vi "Time-calllucated_temp_graph.vi"() -> ()   [LabVIEW 2017]
uses:
  <vilib>/Utility/miscctls.llb/LVCursorListTypeDef.ctl
  <vilib>/measure/NI_MAPro.lvlib
panel:
  out "size(s) 2":i32
  out "Array 11":ext[](array[numeric])
  out "Array 8":timestamp[](array[timestamp])
  out "appended array":timestamp[][](array[timestamp])
  out "deleted portion":ext[](array[numeric])
  out "Array 10":ext[](array[numeric])
  out "Array 9":ext[][](array[numeric])
  out "Array 7":bool[](array[boolean])
  out "output cluster 3":T1(array[cluster])
  in  "Cursor List 3":T2
  out "Numeric 2":i32
  out "Array 6":timestamp[](array[timestamp])
  out "Array 5":dbl[](array[numeric])
  out "Array 4":i32[](array[numeric])
  out "Array 3":u16[](array[numeric])
  out "Array 2":u16[](array[numeric])
  out "Valley Value":dbl[](array[numeric])
  out "Valley Value index":u16[](array[numeric])
  out "Peak Value index":u16[](array[numeric])
  out "Peak Value":dbl[](array[numeric])
  out "# found 2":i32
  in  "peaks/valleys 2":u16(ring)=1 items=["Peaks", "Valleys"]
  out "x = y?":bool
  out "x+y 2":i32
  out "STOP THRESHOLD TRIGGER":i32
  out "START THRESHOLD TRIGGER":i32
  out "Array":timestamp[](array[timestamp])
  out "Numeric":i32
  out "Locations":dbl[](array[numeric]) format="%0.2f"
  out "size(s)":i32
  out "2nd Derivatives":dbl[](array[numeric]) format="%0.2f"
  out "unsigned 16bit integer":u16
  out "output cluster 2":T1(array[cluster])
  in  "Cursor List 2":T2
  out "XY Graph 3":cluster{"X":dbl, "X 2":dbl}[](graph)
  out "element":dbl
  in  "peaks/valleys":u16(ring) items=["Peaks", "Valleys"]
  in  "width":i32=3
  out "# found":i32
  in  "threshold":dbl=130.0 format="%#_13g"
  out "Y":dbl[](array[numeric]) format="%0.2f"
  out "X":dbl[](array[numeric]) format="%0.2f"
  out "time stamp":timestamp[](array[timestamp])
  out "XY Graph 2":cluster{"time stamp":timestamp, "X":dbl}[](graph)
  out "number":ext[](array[numeric])
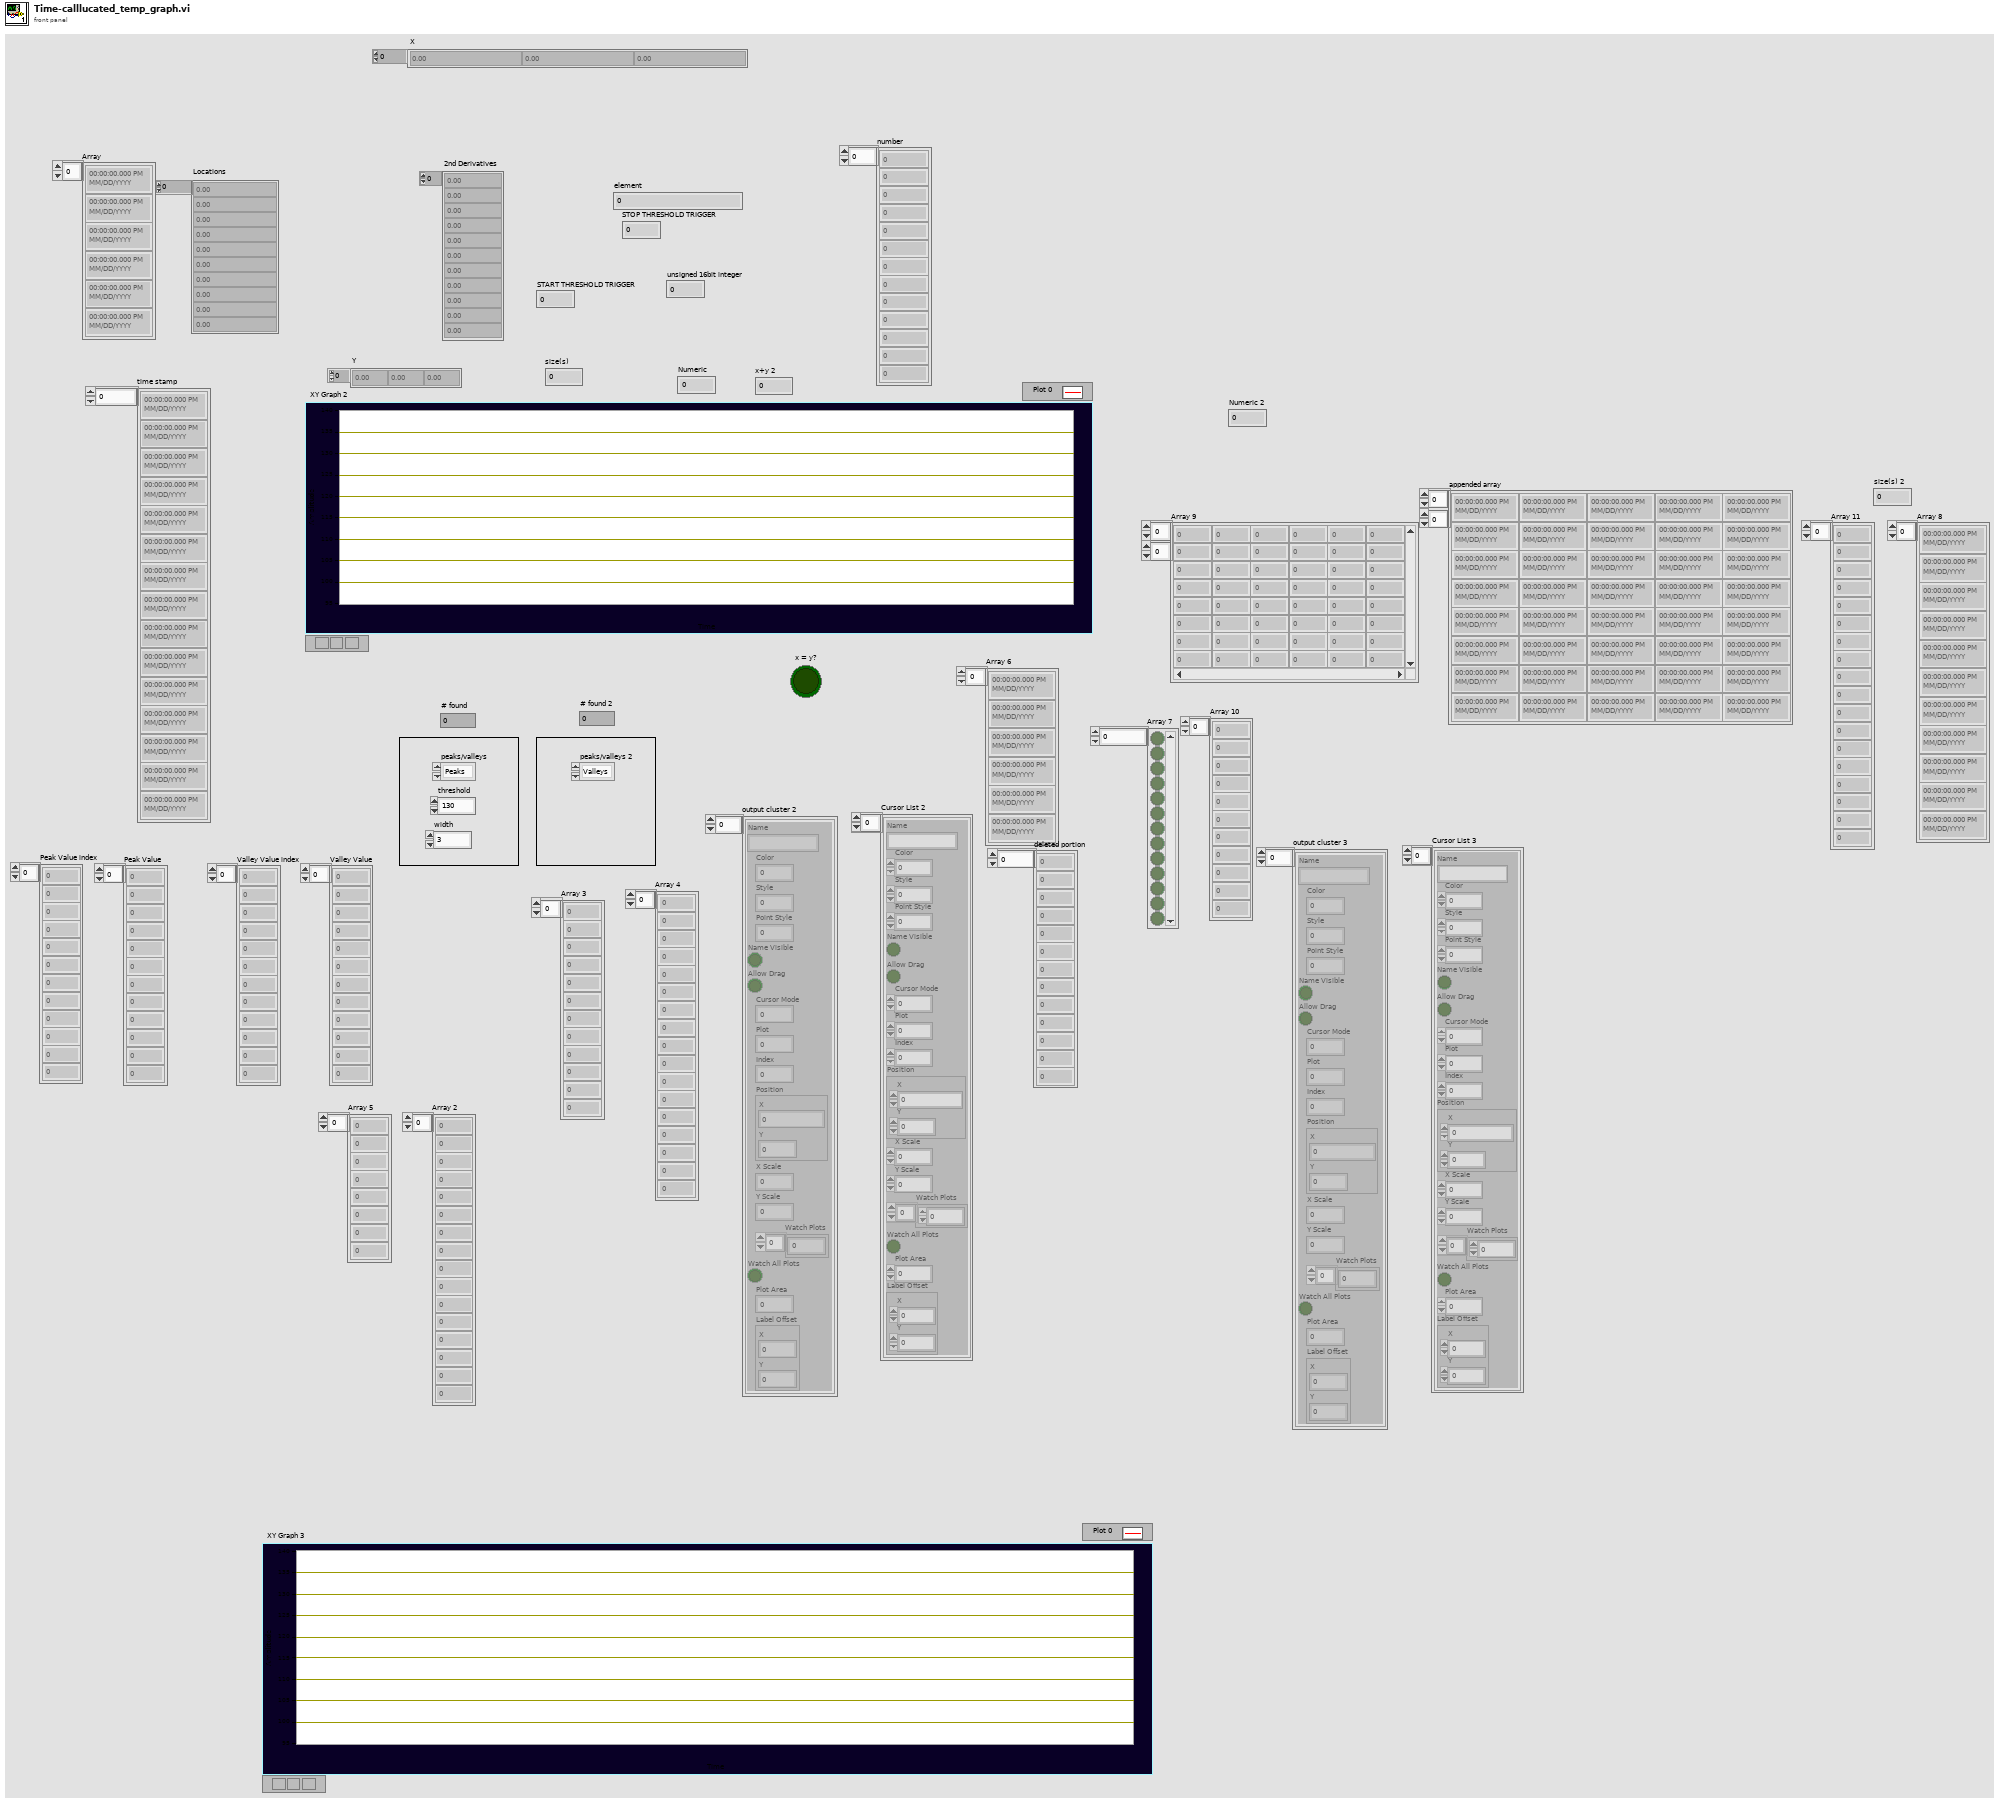
[diagram p1: front panel]
types:
  T1 = cluster{"Name":string, "Color":u32, "Style":u8, "Point Style":u8, "Name Visible":bool, "Allow Drag":bool, "Cursor Mode":u32, "Plot":i32, "Index":i32, "Position":cluster{"X":dbl, "Y":dbl}, "X Scale":u32, "Y Scale":u32, "Watch Plots":i32[], "Watch All Plots":bool, "Plot Area":i32, "Label Offset":cluster{"X":dbl, "Y":dbl}}[]
  T2 = typedef "LVCursorListTypeDef.ctl" = cluster{"Name":string, "Color":u32, "Style":u8, "Point Style":u8, "Name Visible":bool, "Allow Drag":bool, "Cursor Mode":u32, "Plot":i32, "Index":i32, "Position":cluster{"X":dbl, "Y":dbl}, "X Scale":u32, "Y Scale":u32, "Watch Plots":i32[], "Watch All Plots":bool, "Plot Area":i32, "Label Offset":cluster{"X":dbl, "Y":dbl}}[]
  T3 = typedef "LVDateTimeRec.ctl" = cluster{"fractional second":dbl, "second":i32, "minute":i32, "hour":i32, "day of month":i32, "month":i32, "year":i32, "day of week":i32, "day of year":i32, "DST":i32}
  T4 = cluster{"Name":string, "Color":u32, "Style":u8, "Point Style":u8, "Name Visible":bool, "Allow Drag":bool, "Cursor Mode":u32, "Plot":i32, "Index":i32, "Position":cluster{"X":dbl, "Y":dbl}, "X Scale":u32, "Y Scale":u32, "Watch Plots":i32[], "Watch All Plots":bool, "Plot Area":i32, "Label Offset":cluster{"X":dbl, "Y":dbl}}
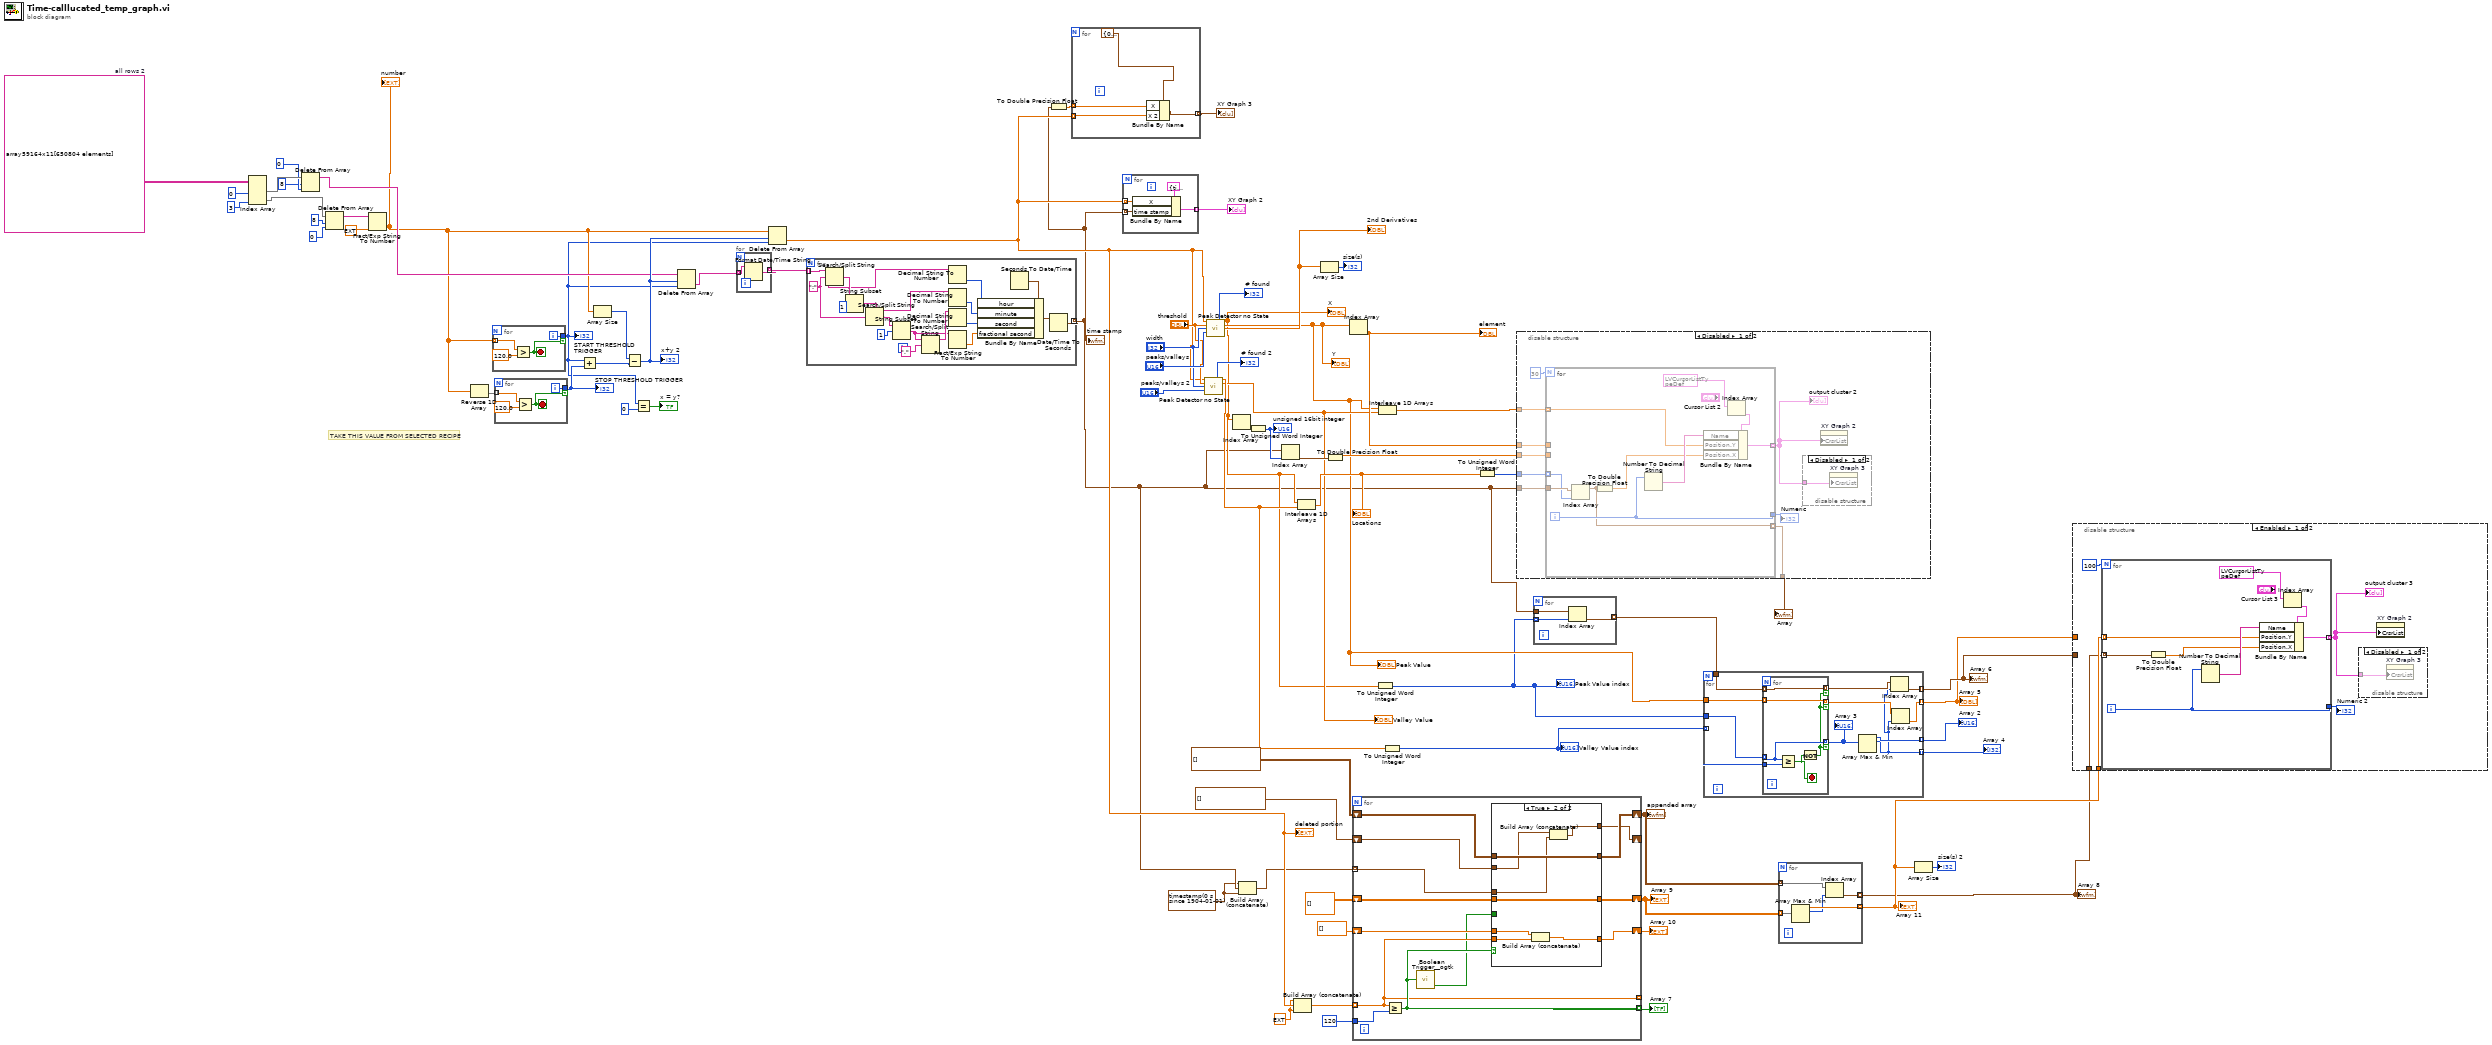
[diagram p0: block diagram]
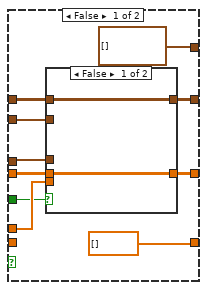
[diagram p2: hidden frame]
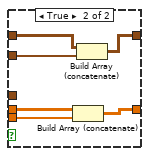
[diagram p3: hidden frame]
diagram:
  w9 = timestamp(0 s since 1904-01-01) ("time stamp")
  w11 = ext 0.0 ("String")
  w67 = string[][] array59164x11[650804 elements]  # all rows 2
  # "TAKE THIS VALUE FROM SELECTED RECIPE"
  n1 = Index Array(array=w67, index (col) #1=0 ("index (row)"), index (col) #2=3 ("disabled index (col)")) -> (element #1=w72:string[], element #2=w68:string[])  [unwired: 2 in]
  n2 = Delete From Array(array=w72, length=8 ("index (row)"), index=0 ("index (row)")) -> (array with subset deleted=w42:string[])  [unwired: 1 out]
  n3 = Delete From Array(array=w68, length=8 ("index (row)"), index=0 ("index (row)")) -> (array with subset deleted=w49:string[])  [unwired: 1 out]
  n4 = Fract/Exp String To Number(string=w49, default (0 dbl)=ext 0.0 ("String")) -> (number=w40:ext[])  [unwired: 2 in, 1 out]
  "number" <- w40
  n5 = Reverse 1D Array(array=w40) -> (reversed array=w48:ext[])
  n6 = for {
    tunnel: w40 -> [w75] mode=indexing
    tunnel: [w74] -> w39 if=w73
    i -> [w74]
    stop <- w73 stop-if-true
    n7 = Greater?(x=w75, y=120.0) -> (0:w73:bool)
  }
  "START THRESHOLD TRIGGER" <- w39
  n8 = for {
    tunnel: w48 -> [w79] mode=indexing
    tunnel: [w78] -> w47 if=w77
    i -> [w78]
    stop <- w77 stop-if-true
    n9 = Greater?(x=w79, y=120.0) -> (0:w77:bool)
  }
  "STOP THRESHOLD TRIGGER" <- w47
  n10 = Add(x=w39, y=w47) -> (x+y=w45:i32)
  n11 = Array Size(array=w40) -> (size(s)=w46:i32)
  n12 = Subtract(x=w46, y=w45) -> (x-y=w44:i32)
  "x+y 2" <- w44
  n13 = Equal?(x=w39, y=0) -> (x = y?=→"x = y?":bool)
  n14 = Delete From Array(array=w42, length=w44, index=w39) -> (deleted portion=w43:string[])  [unwired: 1 out]
  n15 = for {
    tunnel: w43 -> [w82] mode=indexing
    tunnel: [w81] -> w63 mode=indexing
    n16 = Format Date/Time String(time format string (%c)=w82) -> (date/time string=w81:string)  [unwired: 2 in]
  }
  n17 = Delete From Array(array=w40, length=w44, index=w39) -> (deleted portion=w13:ext[])  [unwired: 1 out]
  "deleted portion" <- w13
  n18 = for {
    tunnel: w63 -> [w91] mode=indexing
    tunnel: [w99] -> w10 mode=indexing
    w98 = ":" ("format string")
    n19 = Search/Split String(string=w91, search string/char (-)=w98) -> (substring before match=w87:string, match + rest of string=w96:string)  [unwired: 1 in, 1 out]
    n20 = String Subset(string=w96, offset (0)=1) -> (substring=w95:string)  [unwired: 1 in]
    n21 = Search/Split String(string=w95, search string/char (-)=w98) -> (substring before match=w86:string, match + rest of string=w93:string)  [unwired: 1 in, 1 out]
    n22 = String Subset(string=w93, offset (0)=1) -> (substring=w85:string)  [unwired: 1 in]
    n23 = Search/Split String(string=w85, search string/char (-)="." ("format string")) -> (substring before match=w90:string)  [unwired: 1 in, 2 out]
    n24 = Decimal String To Number(string=w87) -> (number=w88:i32)  [unwired: 2 in, 1 out]
    n25 = Decimal String To Number(string=w86) -> (number=w89:i32)  [unwired: 2 in, 1 out]
    n26 = Decimal String To Number(string=w90) -> (number=w83:i32)  [unwired: 2 in, 1 out]
    n27 = Fract/Exp String To Number(string=w85) -> (number=w84:dbl)  [unwired: 3 in, 1 out]
    n28 = Seconds To Date/Time() -> (date time rec=w100:T3)  [unwired: 2 in]
    n29 = Bundle By Name(cluster=w100, "hour"=w88, "minute"=w89, "second"=w83, "fractional second"=w84) -> (w101:T3)
    n30 = Date/Time To Seconds(2:w101) -> (0:w99:timestamp)  [unwired: 1 in]
  }
  "time stamp" <- w10
  n31 = To Double Precision Float(number=w10) -> (double precision float=w57:dbl[])
  n32 = for {
    tunnel: w57 -> [w103] mode=indexing
    tunnel: [w105] -> w56 mode=indexing
    tunnel: w13 -> [w104] mode=indexing
    n33 = Bundle By Name(cluster=cluster{"X":dbl, "X 2":dbl} {"X"=0.0, "X 2"=0.0}, "X"=w103, "X 2"=w104) -> (w105:cluster{"X":dbl, "X 2":dbl})
  }
  "XY Graph 3" <- w56
  n34 = for {
    tunnel: w13 -> [w106] mode=indexing
    tunnel: [w109] -> w59 mode=indexing
    tunnel: w10 -> [w107] mode=indexing
    n35 = Bundle By Name(cluster=cluster{"time stamp":timestamp, "X":dbl} {"time stamp"=timestamp(0 s since 1904-01-01), "X"=0.0}, "X"=w106, "time stamp"=w107) -> (w109:cluster{"time stamp":timestamp, "X":dbl})
  }
  "XY Graph 2" <- w59
  n36 = call <vilib>:"Peak Detector no State.vi"("X"=w13, "threshold"="threshold", "width"="width", "peaks/valleys"="peaks/valleys 2") -> ("# found"=→"# found 2":i32, "Locations"=w29:dbl[], "Amplitudes"=w28:dbl[])  [unwired: 4 in, 5 out]
  "Valley Value" <- w28
  n37 = call <vilib>:"Peak Detector no State.vi"("X"=w13, "threshold"="threshold", "width"="width", "peaks/valleys"="peaks/valleys") -> ("# found"=→"# found":i32, "Locations"=w19:dbl[], "Amplitudes"=w24:dbl[], "2nd Derivatives"=w52:dbl[])  [unwired: 4 in, 4 out]
  "X" <- w19
  "Y" <- w24
  "2nd Derivatives" <- w52
  "Peak Value" <- w24
  n38 = Index Array(array=w19) -> (element=w55:dbl)  [unwired: 1 in]
  n39 = Build Array (concatenate)(w9, w10, w9) -> (w6:timestamp[])
  n40 = To Unsigned Word Integer(number=w55) -> (unsigned 16bit integer=w54:u16)
  "unsigned 16bit integer" <- w54
  n41 = Index Array(array=w10, index=w54) -> (element=w58:timestamp)
  n42 = Build Array (concatenate)(w11, w13, w11) -> (w12:ext[])
  n43 = Interleave 1D Arrays(w19, w29) -> (w32:dbl[])
  "Locations" <- w32
  n44 = Array Size(array=w52) -> (size(s)=→"size(s)":i32)
  n45 = To Double Precision Float(number=w58) -> (double precision float=w41:dbl)
  n46 = Index Array(array=w24) -> (element=w53:dbl)  [unwired: 1 in]
  "element" <- w53
  n47 = for {
    tunnel: w12 -> [w120] mode=indexing
    tunnel: [w121] -> w17 mode=indexing
    tunnel: 120 -> [w122]
    tunnel: [w120] -> _ mode=indexing
    shift-right: [w119] -> w14
    shift-left: ext[] [] -> [w118]
    shift-right: [w116] -> w5
    shift-left: ext[][] [] -> [w117]
    tunnel: w6 -> [w114] mode=indexing
    shift-right: [w113] -> w4
    shift-left: timestamp[][] [] ("appended array") -> [w112]
    shift-right: [w110] -> _
    shift-left: timestamp[] [] ("appended array") -> [w111]
    n48 = Greater Or Equal?(x=w120, y=w122) -> (x >= y?=w121:bool)
    n49 = call <userlib>:"Boolean Trigger__ogtk.vi"("Boolean Input"=w121) -> ("Falling Edge"=w115:bool)  [unwired: 1 in, 1 out]
    n50 = case shown="True" w121 {
      tunnel: w120 -> [_ w148]
      tunnel: [ext[] [] w147] -> w119
      tunnel: w118 -> [w129 w145]
      tunnel: w117 -> [w130 w146]
      tunnel: [w131 w146] -> w116
      tunnel: w115 -> [w128 _]
      tunnel: w114 -> [w127 w141]
      tunnel: [w126 w144] -> w113
      tunnel: w112 -> [w125 w144]
      tunnel: w111 -> [w124 w142]
      tunnel: [timestamp[] [] ("appended array") w143] -> w110
      frame False {
        n51 = case shown="False" w128 {
          tunnel: [w134 w140] -> w131
          tunnel: w130 -> [w134 w139]
          tunnel: w129 -> [_ w138]
          tunnel: w127 -> [_ _]
          tunnel: [w133 w137] -> w126
          tunnel: w125 -> [w133 w136]
          tunnel: w124 -> [_ w135]
          frame False {
          }
          frame True {
            n52 = Build Array (concatenate)(w139, w138) -> (w140:ext[][])
            n53 = Build Array (concatenate)(w136, w135) -> (w137:timestamp[][])
          }
        }
      }
      frame True {
        n54 = Build Array (concatenate)(w145, w148) -> (w147:ext[])
        n55 = Build Array (concatenate)(w142, w141) -> (w143:timestamp[])
      }
    }
  }
  "Array 7" <- w17
  "Array 9" <- w5
  "Array 10" <- w14
  "appended array" <- w4
  n56 = To Unsigned Word Integer(number=w19) -> (unsigned 16bit integer=w21:u16[])
  "Peak Value index" <- w21
  n57 = Interleave 1D Arrays(w24, w28) -> (w31:dbl[])
  n58 = To Unsigned Word Integer(number=w29) -> (unsigned 16bit integer=w27:u16[])
  "Valley Value index" <- w27
  n59 = To Unsigned Word Integer(number=w32) -> (unsigned 16bit integer=w30:u16[])
  n60 = disable-structure shown="Disabled" {
    disable-tunnel: w41 -> [w157 _]
    disable-tunnel: w53 -> [w156 _]
    disable-tunnel: w31 -> [w150 _]
    disable-tunnel: w10 -> [w155 _]
    disable-tunnel: w30 -> [w149 _]
    disable-tunnel: [w153 _] -> w50
    frame Disabled {
      n61 = for {
        N: 30 -> [_]
        tunnel: [w167] -> w151 mode=indexing
        tunnel: w157 -> [_]
        tunnel: w156 -> [_]
        tunnel: w150 -> [w165] mode=indexing
        tunnel: w155 -> [w163]
        tunnel: w149 -> [w162] mode=indexing
        tunnel: [w161] -> w154
        tunnel: [w160] -> w153 mode=indexing
        i -> [w161]
        n62 = Index Array(array=w163, index=w162) -> (element=w160:timestamp)
        n63 = To Double Precision Float(number=w160) -> (double precision float=w164:dbl)
        n64 = Number To Decimal String(number=w161) -> (decimal integer string=w166:string)  [unwired: 1 in]
        n65 = Index Array(array=T2 [{"Name"="0", "Color"=0, "Style"=0, "Point Style"=13, "Name Visible"=FALSE, "Allow Drag"=FALSE, "Cursor Mode"=0, "Plot"=0, "Index"=0, "Position"={"X"=3725289003.72, "Y"=121.765}, "X Scale"=0, "Y Scale"=0, "Watch Plots"=[], "Watch All Plots"=FALSE, "Plot Area"=0, "Label Offset"={"X"=0.0, "Y"=0.0}}, {"Name"="1", "Color"=0, "Style"=0, "Point Style"=0, "Name Visible"=FALSE, "Allow Drag"=FALSE, "Cursor Mode"=0, "Plot"=0, "Index"=0, "Position"={"X"=3725289003.725, "Y"=125.02090909090909}, "X Scale"=0, "Y Scale"=0, "Watch Plots"=[], "Watch All Plots"=FALSE, "Plot Area"=0, "Label Offset"={"X"=0.0, "Y"=0.0}}, {"Name"="2", "Color"=0, "Style"=0, "Point Style"=0, "Name Visible"=FALSE, "Allow Drag"=FALSE, "Cursor Mode"=0, "Plot"=0, "Index"=0, "Position"={"X"=3725289003.728, "Y"=128.01}, "X Scale"=0, "Y Scale"=0, "Watch Plots"=[], "Watch All Plots"=FALSE, "Plot Area"=0, "Label Offset"={"X"=0.0, "Y"=0.0}}, {"Name"="3", "Color"=0, "Style"=0, "Point Style"=0, "Name Visible"=FALSE, "Allow Drag"=FALSE, "Cursor Mode"=0, "Plot"=0, "Index"=0, "Position"={"X"=3725289003.73, "Y"=123.4901219512195}, "X Scale"=0, "Y Scale"=0, "Watch Plots"=[], "Watch All Plots"=FALSE, "Plot Area"=0, "Label Offset"={"X"=0.0, "Y"=0.0}}, {"Name"="4", "Color"=0, "Style"=0, "Point Style"=0, "Name Visible"=FALSE, "Allow Drag"=FALSE, "Cursor Mode"=0, "Plot"=0, "Index"=0, "Position"={"X"=3725289003.732, "Y"=120.435}, "X Scale"=0, "Y Scale"=0, "Watch Plots"=[], "Watch All Plots"=FALSE, "Plot Area"=0, "Label Offset"={"X"=0.0, "Y"=0.0}}, {"Name"="5", "Color"=0, "Style"=0, "Point Style"=0, "Name Visible"=FALSE, "Allow Drag"=FALSE, "Cursor Mode"=0, "Plot"=0, "Index"=0, "Position"={"X"=3725289003.752, "Y"=121.25480392156864}, "X Scale"=0, "Y Scale"=0, "Watch Plots"=[], "Watch All Plots"=FALSE, "Plot Area"=0, "Label Offset"={"X"=0.0, "Y"=0.0}}, {"Name"="6", "Color"=0, "Style"=0, "Point Style"=0, "Name Visible"=FALSE, "Allow Drag"=FALSE, "Cursor Mode"=0, "Plot"=0, "Index"=0, "Position"={"X"=3725289003.756, "Y"=123.92999999999999}, "X Scale"=0, "Y Scale"=0, "Watch Plots"=[], "Watch All Plots"=FALSE, "Plot Area"=0, "Label Offset"={"X"=0.0, "Y"=0.0}}, {"Name"="7", "Color"=0, "Style"=0, "Point Style"=0, "Name Visible"=FALSE, "Allow Drag"=FALSE, "Cursor Mode"=0, "Plot"=0, "Index"=0, "Position"={"X"=3725289003.762, "Y"=127.01970588235294}, "X Scale"=0, "Y Scale"=0, "Watch Plots"=[], "Watch All Plots"=FALSE, "Plot Area"=0, "Label Offset"={"X"=0.0, "Y"=0.0}}, {"Name"="8", "Color"=0, "Style"=0, "Point Style"=0, "Name Visible"=FALSE, "Allow Drag"=FALSE, "Cursor Mode"=0, "Plot"=0, "Index"=0, "Position"={"X"=3725289003.765, "Y"=131.29425531914893}, "X Scale"=0, "Y Scale"=0, "Watch Plots"=[], "Watch All Plots"=FALSE, "Plot Area"=0, "Label Offset"={"X"=0.0, "Y"=0.0}}, {"Name"="9", "Color"=0, "Style"=0, "Point Style"=0, "Name Visible"=FALSE, "Allow Drag"=FALSE, "Cursor Mode"=0, "Plot"=0, "Index"=0, "Position"={"X"=3725289003.767, "Y"=128.4116891891892}, "X Scale"=0, "Y Scale"=0, "Watch Plots"=[], "Watch All Plots"=FALSE, "Plot Area"=0, "Label Offset"={"X"=0.0, "Y"=0.0}}, {"Name"="10", "Color"=0, "Style"=0, "Point Style"=0, "Name Visible"=FALSE, "Allow Drag"=FALSE, "Cursor Mode"=0, "Plot"=0, "Index"=0, "Position"={"X"=3725289003.768, "Y"=122.84}, "X Scale"=0, "Y Scale"=0, "Watch Plots"=[], "Watch All Plots"=FALSE, "Plot Area"=0, "Label Offset"={"X"=0.0, "Y"=0.0}}, {"Name"="11", "Color"=0, "Style"=0, "Point Style"=0, "Name Visible"=FALSE, "Allow Drag"=FALSE, "Cursor Mode"=0, "Plot"=0, "Index"=0, "Position"={"X"=3725289003.794, "Y"=121.99}, "X Scale"=0, "Y Scale"=0, "Watch Plots"=[], "Watch All Plots"=FALSE, "Plot Area"=0, "Label Offset"={"X"=0.0, "Y"=0.0}}, {"Name"="12", "Color"=0, "Style"=0, "Point Style"=0, "Name Visible"=FALSE, "Allow Drag"=FALSE, "Cursor Mode"=0, "Plot"=0, "Index"=0, "Position"={"X"=3725289003.803, "Y"=128.6199504950495}, "X Scale"=0, "Y Scale"=0, "Watch Plots"=[], "Watch All Plots"=FALSE, "Plot Area"=0, "Label Offset"={"X"=0.0, "Y"=0.0}}, {"Name"="13", "Color"=0, "Style"=0, "Point Style"=0, "Name Visible"=FALSE, "Allow Drag"=FALSE, "Cursor Mode"=0, "Plot"=0, "Index"=0, "Position"={"X"=3725289003.806, "Y"=132.86499999999998}, "X Scale"=0, "Y Scale"=0, "Watch Plots"=[], "Watch All Plots"=FALSE, "Plot Area"=0, "Label Offset"={"X"=0.0, "Y"=0.0}}, {"Name"="14", "Color"=0, "Style"=0, "Point Style"=0, "Name Visible"=FALSE, "Allow Drag"=FALSE, "Cursor Mode"=0, "Plot"=0, "Index"=0, "Position"={"X"=3725289003.808, "Y"=128.93437743190663}, "X Scale"=0, "Y Scale"=0, "Watch Plots"=[], "Watch All Plots"=FALSE, "Plot Area"=0, "Label Offset"={"X"=0.0, "Y"=0.0}}, {"Name"="15", "Color"=0, "Style"=0, "Point Style"=0, "Name Visible"=FALSE, "Allow Drag"=FALSE, "Cursor Mode"=0, "Plot"=0, "Index"=0, "Position"={"X"=3725289003.83, "Y"=121.8}, "X Scale"=0, "Y Scale"=0, "Watch Plots"=[], "Watch All Plots"=FALSE, "Plot Area"=0, "Label Offset"={"X"=0.0, "Y"=0.0}}, {"Name"="16", "Color"=0, "Style"=0, "Point Style"=0, "Name Visible"=FALSE, "Allow Drag"=FALSE, "Cursor Mode"=0, "Plot"=0, "Index"=0, "Position"={"X"=3725289003.84, "Y"=128.54500000000002}, "X Scale"=0, "Y Scale"=0, "Watch Plots"=[], "Watch All Plots"=FALSE, "Plot Area"=0, "Label Offset"={"X"=0.0, "Y"=0.0}}, {"Name"="17", "Color"=0, "Style"=0, "Point Style"=0, "Name Visible"=FALSE, "Allow Drag"=FALSE, "Cursor Mode"=0, "Plot"=0, "Index"=0, "Position"={"X"=3725289003.842, "Y"=129.14884615384614}, "X Scale"=0, "Y Scale"=0, "Watch Plots"=[], "Watch All Plots"=FALSE, "Plot Area"=0, "Label Offset"={"X"=0.0, "Y"=0.0}}, {"Name"="18", "Color"=0, "Style"=0, "Point Style"=0, "Name Visible"=FALSE, "Allow Drag"=FALSE, "Cursor Mode"=0, "Plot"=0, "Index"=0, "Position"={"X"=3725289003.845, "Y"=133.010296912114}, "X Scale"=0, "Y Scale"=0, "Watch Plots"=[], "Watch All Plots"=FALSE, "Plot Area"=0, "Label Offset"={"X"=0.0, "Y"=0.0}}, {"Name"="19", "Color"=0, "Style"=0, "Point Style"=0, "Name Visible"=FALSE, "Allow Drag"=FALSE, "Cursor Mode"=0, "Plot"=0, "Index"=0, "Position"={"X"=3725289003.847, "Y"=128.22329145728645}, "X Scale"=0, "Y Scale"=0, "Watch Plots"=[], "Watch All Plots"=FALSE, "Plot Area"=0, "Label Offset"={"X"=0.0, "Y"=0.0}}] ("Cursor List")) -> (element=w168:T4)  [unwired: 1 in]
        n66 = Bundle By Name(cluster=w168, "Name"=w166, "Position.Y"=w165, "Position.X"=w164) -> (w167:T4)
      }
      "output cluster 2" <- w151
      "Numeric" <- w154
      n67 = disable-structure shown="Disabled" {
        disable-tunnel: w151 -> [w158 _]
        frame Disabled {
          n68 = property on="XY Graph 3" class="XYGraph (strict)"("CrsrList"=w158) -> ()  [unwired: 2 in, 2 out]
        }
        frame Enabled {
        }
      }
      n69 = property on="XY Graph 2" class="XYGraph (strict)"("CrsrList"=w151) -> ()  [unwired: 2 in, 2 out]
    }
    frame Enabled {
    }
  }
  "Array" <- w50
  n70 = for {
    tunnel: w10 -> [w171]
    tunnel: w21 -> [w170] mode=indexing
    tunnel: [w169] -> w20 mode=indexing
    n71 = Index Array(array=w171, index=w170) -> (element=w169:timestamp)
  }
  n72 = for {
    tunnel: w27 -> [w181] mode=indexing
    tunnel: w21 -> [w182]
    tunnel: [w179] -> w26 mode=indexing
    tunnel: [w173] -> w25 mode=indexing
    tunnel: w24 -> [w178]
    tunnel: [w176] -> w22 mode=indexing
    tunnel: w20 -> [w175]
    tunnel: [w172] -> w23 mode=indexing
    n73 = for {
      tunnel: w181 -> [w188]
      tunnel: w182 -> [w187] mode=indexing
      tunnel: [w187] -> w180 mode=indexing if=w183
      tunnel: [w185] -> w177 mode=indexing if=w183
      tunnel: w178 -> [w185] mode=indexing
      tunnel: w175 -> [w184] mode=indexing
      tunnel: [w184] -> w174 mode=indexing if=w183
      stop <- w186 stop-if-true
      n74 = Greater Or Equal?(x=w187, y=w188) -> (x >= y?=w186:bool)
      n75 = Not(x=w186) -> (.not. x?=w183:bool)
    }
    "Array 3" <- w180
    n76 = Array Max & Min(array=w180) -> (max value=w179:u16, max index (indices)=w173:i32)  [unwired: 2 out]
    n77 = Index Array(array=w174, index=w173) -> (element=w172:timestamp)
    n78 = Index Array(array=w177, index=w173) -> (element=w176:dbl)
  }
  "Array 2" <- w26
  "Array 4" <- w25
  "Array 5" <- w22
  "Array 6" <- w23
  n79 = for {
    tunnel: w5 -> [w193] mode=indexing
    tunnel: w4 -> [w191] mode=indexing
    tunnel: [w192] -> w2 mode=indexing
    tunnel: [w189] -> w1 mode=indexing
    n80 = Array Max & Min(array=w193) -> (max value=w192:ext, max index (indices)=w190:i32)  [unwired: 2 out]
    n81 = Index Array(array=w191, index=w190) -> (element=w189:timestamp)
  }
  "Array 8" <- w1
  "Array 11" <- w2
  n82 = Array Size(array=w2) -> (size(s)=→"size(s) 2":i32)
  n83 = disable-structure shown="Enabled" {
    disable-tunnel: w23 -> [_ _]
    disable-tunnel: w22 -> [_ _]
    disable-tunnel: w2 -> [w195 _]
    disable-tunnel: w1 -> [w194 _]
    frame Enabled {
      n84 = for {
        N: 100 -> [_]
        tunnel: [w206] -> w196 mode=indexing
        tunnel: [w203] -> w198
        tunnel: w194 -> [w201] mode=indexing
        tunnel: w195 -> [w200] mode=indexing
        i -> [w203]
        n85 = To Double Precision Float(number=w201) -> (double precision float=w204:dbl)
        n86 = Number To Decimal String(number=w203) -> (decimal integer string=w205:string)  [unwired: 1 in]
        n87 = Index Array(array=T2 [{"Name"="0", "Color"=0, "Style"=0, "Point Style"=13, "Name Visible"=FALSE, "Allow Drag"=FALSE, "Cursor Mode"=0, "Plot"=0, "Index"=0, "Position"={"X"=3725289003.72, "Y"=121.765}, "X Scale"=0, "Y Scale"=0, "Watch Plots"=[], "Watch All Plots"=FALSE, "Plot Area"=0, "Label Offset"={"X"=0.0, "Y"=0.0}}, {"Name"="1", "Color"=0, "Style"=0, "Point Style"=0, "Name Visible"=FALSE, "Allow Drag"=FALSE, "Cursor Mode"=0, "Plot"=0, "Index"=0, "Position"={"X"=3725289003.725, "Y"=125.02090909090909}, "X Scale"=0, "Y Scale"=0, "Watch Plots"=[], "Watch All Plots"=FALSE, "Plot Area"=0, "Label Offset"={"X"=0.0, "Y"=0.0}}, {"Name"="2", "Color"=0, "Style"=0, "Point Style"=0, "Name Visible"=FALSE, "Allow Drag"=FALSE, "Cursor Mode"=0, "Plot"=0, "Index"=0, "Position"={"X"=3725289003.728, "Y"=128.01}, "X Scale"=0, "Y Scale"=0, "Watch Plots"=[], "Watch All Plots"=FALSE, "Plot Area"=0, "Label Offset"={"X"=0.0, "Y"=0.0}}, {"Name"="3", "Color"=0, "Style"=0, "Point Style"=0, "Name Visible"=FALSE, "Allow Drag"=FALSE, "Cursor Mode"=0, "Plot"=0, "Index"=0, "Position"={"X"=3725289003.73, "Y"=123.4901219512195}, "X Scale"=0, "Y Scale"=0, "Watch Plots"=[], "Watch All Plots"=FALSE, "Plot Area"=0, "Label Offset"={"X"=0.0, "Y"=0.0}}, {"Name"="4", "Color"=0, "Style"=0, "Point Style"=0, "Name Visible"=FALSE, "Allow Drag"=FALSE, "Cursor Mode"=0, "Plot"=0, "Index"=0, "Position"={"X"=3725289003.732, "Y"=120.435}, "X Scale"=0, "Y Scale"=0, "Watch Plots"=[], "Watch All Plots"=FALSE, "Plot Area"=0, "Label Offset"={"X"=0.0, "Y"=0.0}}, {"Name"="5", "Color"=0, "Style"=0, "Point Style"=0, "Name Visible"=FALSE, "Allow Drag"=FALSE, "Cursor Mode"=0, "Plot"=0, "Index"=0, "Position"={"X"=3725289003.752, "Y"=121.25480392156864}, "X Scale"=0, "Y Scale"=0, "Watch Plots"=[], "Watch All Plots"=FALSE, "Plot Area"=0, "Label Offset"={"X"=0.0, "Y"=0.0}}, {"Name"="6", "Color"=0, "Style"=0, "Point Style"=0, "Name Visible"=FALSE, "Allow Drag"=FALSE, "Cursor Mode"=0, "Plot"=0, "Index"=0, "Position"={"X"=3725289003.756, "Y"=123.92999999999999}, "X Scale"=0, "Y Scale"=0, "Watch Plots"=[], "Watch All Plots"=FALSE, "Plot Area"=0, "Label Offset"={"X"=0.0, "Y"=0.0}}, {"Name"="7", "Color"=0, "Style"=0, "Point Style"=0, "Name Visible"=FALSE, "Allow Drag"=FALSE, "Cursor Mode"=0, "Plot"=0, "Index"=0, "Position"={"X"=3725289003.762, "Y"=127.01970588235294}, "X Scale"=0, "Y Scale"=0, "Watch Plots"=[], "Watch All Plots"=FALSE, "Plot Area"=0, "Label Offset"={"X"=0.0, "Y"=0.0}}, {"Name"="8", "Color"=0, "Style"=0, "Point Style"=0, "Name Visible"=FALSE, "Allow Drag"=FALSE, "Cursor Mode"=0, "Plot"=0, "Index"=0, "Position"={"X"=3725289003.765, "Y"=131.29425531914893}, "X Scale"=0, "Y Scale"=0, "Watch Plots"=[], "Watch All Plots"=FALSE, "Plot Area"=0, "Label Offset"={"X"=0.0, "Y"=0.0}}, {"Name"="9", "Color"=0, "Style"=0, "Point Style"=0, "Name Visible"=FALSE, "Allow Drag"=FALSE, "Cursor Mode"=0, "Plot"=0, "Index"=0, "Position"={"X"=3725289003.767, "Y"=128.4116891891892}, "X Scale"=0, "Y Scale"=0, "Watch Plots"=[], "Watch All Plots"=FALSE, "Plot Area"=0, "Label Offset"={"X"=0.0, "Y"=0.0}}, {"Name"="10", "Color"=0, "Style"=0, "Point Style"=0, "Name Visible"=FALSE, "Allow Drag"=FALSE, "Cursor Mode"=0, "Plot"=0, "Index"=0, "Position"={"X"=3725289003.768, "Y"=122.84}, "X Scale"=0, "Y Scale"=0, "Watch Plots"=[], "Watch All Plots"=FALSE, "Plot Area"=0, "Label Offset"={"X"=0.0, "Y"=0.0}}, {"Name"="11", "Color"=0, "Style"=0, "Point Style"=0, "Name Visible"=FALSE, "Allow Drag"=FALSE, "Cursor Mode"=0, "Plot"=0, "Index"=0, "Position"={"X"=3725289003.794, "Y"=121.99}, "X Scale"=0, "Y Scale"=0, "Watch Plots"=[], "Watch All Plots"=FALSE, "Plot Area"=0, "Label Offset"={"X"=0.0, "Y"=0.0}}, {"Name"="12", "Color"=0, "Style"=0, "Point Style"=0, "Name Visible"=FALSE, "Allow Drag"=FALSE, "Cursor Mode"=0, "Plot"=0, "Index"=0, "Position"={"X"=3725289003.803, "Y"=128.6199504950495}, "X Scale"=0, "Y Scale"=0, "Watch Plots"=[], "Watch All Plots"=FALSE, "Plot Area"=0, "Label Offset"={"X"=0.0, "Y"=0.0}}, {"Name"="13", "Color"=0, "Style"=0, "Point Style"=0, "Name Visible"=FALSE, "Allow Drag"=FALSE, "Cursor Mode"=0, "Plot"=0, "Index"=0, "Position"={"X"=3725289003.806, "Y"=132.86499999999998}, "X Scale"=0, "Y Scale"=0, "Watch Plots"=[], "Watch All Plots"=FALSE, "Plot Area"=0, "Label Offset"={"X"=0.0, "Y"=0.0}}, {"Name"="14", "Color"=0, "Style"=0, "Point Style"=0, "Name Visible"=FALSE, "Allow Drag"=FALSE, "Cursor Mode"=0, "Plot"=0, "Index"=0, "Position"={"X"=3725289003.808, "Y"=128.93437743190663}, "X Scale"=0, "Y Scale"=0, "Watch Plots"=[], "Watch All Plots"=FALSE, "Plot Area"=0, "Label Offset"={"X"=0.0, "Y"=0.0}}, {"Name"="15", "Color"=0, "Style"=0, "Point Style"=0, "Name Visible"=FALSE, "Allow Drag"=FALSE, "Cursor Mode"=0, "Plot"=0, "Index"=0, "Position"={"X"=3725289003.83, "Y"=121.8}, "X Scale"=0, "Y Scale"=0, "Watch Plots"=[], "Watch All Plots"=FALSE, "Plot Area"=0, "Label Offset"={"X"=0.0, "Y"=0.0}}, {"Name"="16", "Color"=0, "Style"=0, "Point Style"=0, "Name Visible"=FALSE, "Allow Drag"=FALSE, "Cursor Mode"=0, "Plot"=0, "Index"=0, "Position"={"X"=3725289003.84, "Y"=128.54500000000002}, "X Scale"=0, "Y Scale"=0, "Watch Plots"=[], "Watch All Plots"=FALSE, "Plot Area"=0, "Label Offset"={"X"=0.0, "Y"=0.0}}, {"Name"="17", "Color"=0, "Style"=0, "Point Style"=0, "Name Visible"=FALSE, "Allow Drag"=FALSE, "Cursor Mode"=0, "Plot"=0, "Index"=0, "Position"={"X"=3725289003.842, "Y"=129.14884615384614}, "X Scale"=0, "Y Scale"=0, "Watch Plots"=[], "Watch All Plots"=FALSE, "Plot Area"=0, "Label Offset"={"X"=0.0, "Y"=0.0}}, {"Name"="18", "Color"=0, "Style"=0, "Point Style"=0, "Name Visible"=FALSE, "Allow Drag"=FALSE, "Cursor Mode"=0, "Plot"=0, "Index"=0, "Position"={"X"=3725289003.845, "Y"=133.010296912114}, "X Scale"=0, "Y Scale"=0, "Watch Plots"=[], "Watch All Plots"=FALSE, "Plot Area"=0, "Label Offset"={"X"=0.0, "Y"=0.0}}, {"Name"="19", "Color"=0, "Style"=0, "Point Style"=0, "Name Visible"=FALSE, "Allow Drag"=FALSE, "Cursor Mode"=0, "Plot"=0, "Index"=0, "Position"={"X"=3725289003.847, "Y"=128.22329145728645}, "X Scale"=0, "Y Scale"=0, "Watch Plots"=[], "Watch All Plots"=FALSE, "Plot Area"=0, "Label Offset"={"X"=0.0, "Y"=0.0}}] ("Cursor List")) -> (element=w207:T4)  [unwired: 1 in]
        n88 = Bundle By Name(cluster=w207, "Name"=w205, "Position.Y"=w200, "Position.X"=w204) -> (w206:T4)
      }
      "output cluster 3" <- w196
      "Numeric 2" <- w198
      n89 = disable-structure shown="Disabled" {
        disable-tunnel: w196 -> [w199 _]
        frame Disabled {
          n90 = property on="XY Graph 3" class="XYGraph (strict)"("CrsrList"=w199) -> ()  [unwired: 2 in, 2 out]
        }
        frame Enabled {
        }
      }
      n91 = property on="XY Graph 2" class="XYGraph (strict)"("CrsrList"=w196) -> ()  [unwired: 2 in, 2 out]
    }
    frame Disabled {
    }
  }
